vi "MALT132 get one output.vi"() -> ()   [LabVIEW 2018]
uses:
  <instrlib>/AltonTech MALT/AltonTech MALT200817.lvlib
panel:
  in  "Address":i32=12 format="%02x"
  in  "Kn":i32=1
  out "Kn Status":bool
  in  "stop":bool
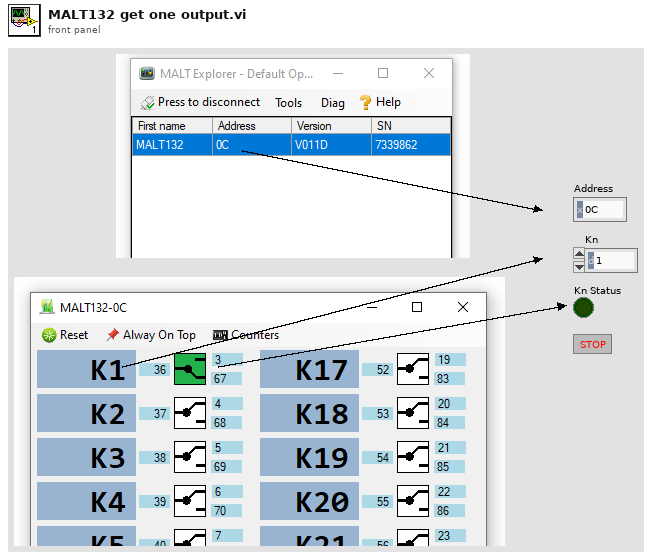
[diagram p1: front panel]
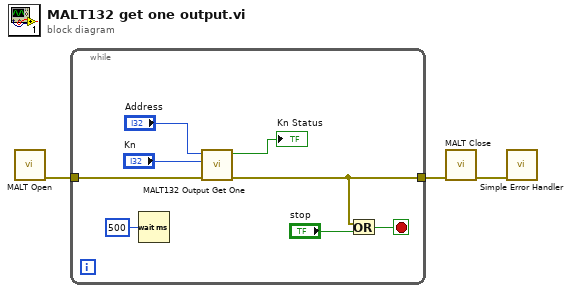
[diagram p0: block diagram]
diagram:
  n1 = call <instrlib>:"MALT Open.vi"() -> ("error out"=w3:errorcluster)  [unwired: 10 in, 1 out]
  n2 = while {
    tunnel: w3 -> [w11]
    tunnel: [w7] -> w2
    stop <- w8 stop-if-true
    n3 = Wait (ms)(milliseconds to wait=u32 500) -> ()  [unwired: 1 out]
    n4 = call <instrlib>:"MALT132 Output Get One.vi"("error in"=w11, "Kn"="Kn", "Address"="Address") -> ("error out"=w7:errorcluster, "status"=→"Kn Status":bool)  [unwired: 7 in]
    n5 = Or(x=w7, y="stop") -> (x .or. y?=w8:bool)
  }
  n6 = call <instrlib>:"MALT Close.vi"("error in"=w2) -> ("error out"=w1:errorcluster)  [unwired: 10 in]
  n7 = call <vilib>:"Simple Error Handler.vi"("error in (no error)"=w1) -> ()  [unwired: 4 in, 5 out]
